vi "TCP Scanner.vi"(3 "Port（4001）":u16=4001, 4 "byte of read(9)":i32=9, 5 "ip":string) -> (0 "status":bool, 1 "错误输出":errorcluster, 2 "Barcode":string)   [LabVIEW 2014]
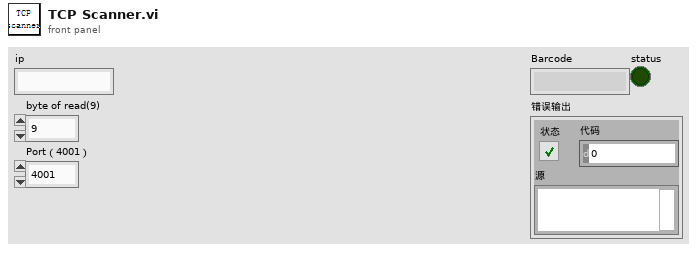
[diagram p1: front panel]
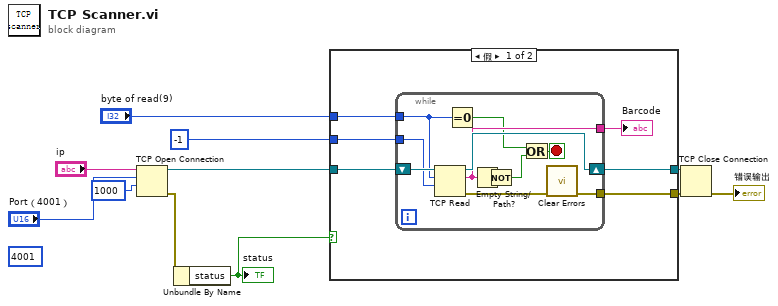
[diagram p0: block diagram]
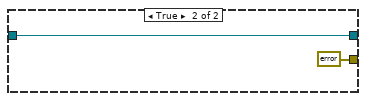
[diagram p2: hidden frame]
diagram:
  (unwired) u16 4001 ("远程端口或服务名称")
  n1 = TCP Open Connection(address="ip", remote port or service name="Port（4001）", timeout ms (60000)=1000 ("超时毫秒(60000)")) -> (connection ID=w10:refnum<k5>, error out=w2:errorcluster)  [unwired: 2 in]
  n2 = Unbundle By Name(w2) -> ("status"=w1:bool)
  "status" <- w1
  n3 = case shown="假" w1 {
    tunnel: w10 -> [w16 w30]
    tunnel: [w15 w30] -> w9
    tunnel: [w14 errorcluster {"status"=FALSE, "code"=0, "source"=""} ("error out")] -> w8
    tunnel: -1 ("超时毫秒(25000)") -> [w13 _]
    tunnel: "byte of read(9)" -> [w12 _]
    frame False {
      n4 = while {
        tunnel: [w23] -> w17
        tunnel: w13 -> [w26]
        tunnel: w12 -> [w21]
        shift-right: [w27] -> w15
        shift-left: w16 -> [w28]
        tunnel: [w24] -> w14
        stop <- w18 stop-if-true
        n5 = TCP Read(connection ID=w28, bytes to read=w21, 9:w26) -> (connection ID out=w27:refnum<k5>, data out=w23:string, error out=w25:errorcluster)  [unwired: 2 in]
        n6 = Equal To 0?(x=w21) -> (x = 0?=w19:bool)
        n7 = Empty String/Path?(string/path=w23) -> (empty?=w22:bool)
        n8 = Not(x=w22) -> (.not. x?=w20:bool)
        n9 = Or(x=w19, y=w20) -> (x .or. y?=w18:bool)
        n10 = call <vilib>:"Clear Errors.vi"("error in (no error)"=w25) -> ("error out"=w24:errorcluster)  [unwired: 5 in, 1 out]
      }
      "Barcode" <- w17
    }
    frame True {
    }
  }
  n11 = TCP Close Connection(connection ID=w9, error in (no error)=w8) -> (error out=→"错误输出":errorcluster)  [unwired: 1 in, 1 out]
